vi "isReporting.vi"(8 "error in (no error)":errorcluster, 11 "Test Report.Default in":refnum<class "Test Report.Event.lvclass">) -> (0 "error out":errorcluster, 2 "Exporting?":bool, 3 "Test Report.Default out":refnum<class "Test Report.Event.lvclass">)   [LabVIEW 2013, in "Caraya.lvlib" / "Test Report.Event.lvclass"]
uses:
  Test Report.Event.lvclass
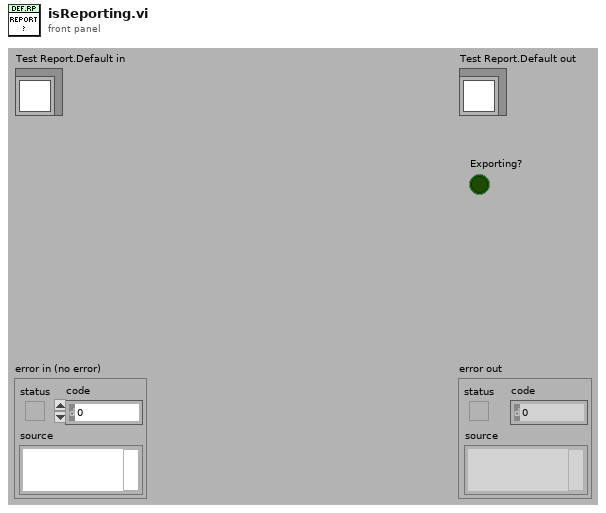
[diagram p1: front panel]
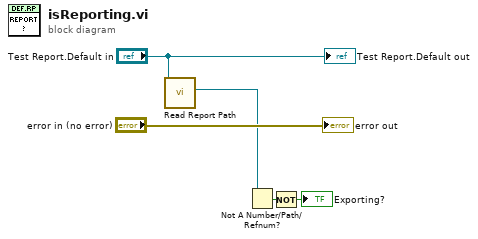
[diagram p0: block diagram]
diagram:
  n1 = call "Read Report Path.vi"("Test Report.Default in"="Test Report.Default in") -> ("Report Event"=w2:refnum<user-event>)  [unwired: 9 in, 1 out]
  n2 = Not A Number/Path/Refnum?(number/path/refnum=w2) -> (NaN/Path/Refnum?=w3:bool)
  n3 = Not(x=w3) -> (.not. x?=→"Exporting?":bool)
  "error out" <- "error in (no error)"
  "Test Report.Default out" <- "Test Report.Default in"
